vi "Close.vi"(8 "error in (no error)":errorcluster, 11 "FPGA Interface in":refnum<class "FPGA Interface.lvclass">) -> (0 "error out":errorcluster)   [LabVIEW 2020, in "BCI-1553 API.lvlib" / "FPGA Interface.lvlib" / "FPGA Interface.lvclass"]
doc: "Ends the FPGA session that is supporting the communication with the BCI-1553 modules."
uses:
  FPGA Interface.lvclass
  FPGA Interface.lvclass/FPGA Interface.ctl
  <vilib>/FPGAPlugInAG/Dynamic/niLvFpga_Close_Dynamic.vi
  <vilib>/rvi/interface/nirviCloseFPGA/nirviCloseFPGA.xnode
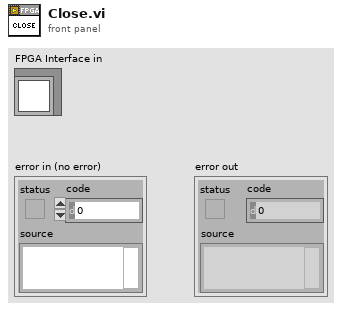
[diagram p1: front panel]
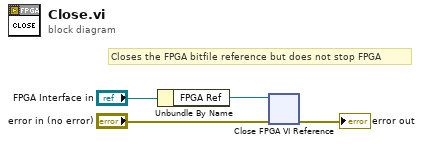
[diagram p0: block diagram]
diagram:
  # "Closes the FPGA bitfile reference but does not stop FPGA"
  n1 = Unbundle By Name("FPGA Interface in") -> ("FPGA Ref"=w1:refnum<k20>)
  n2 = xnode "Close FPGA VI Reference"("FPGA VI Reference In"=w1, "error in"="error in (no error)") -> ("error out"=→"error out":errorcluster)
